vi "恢复参数.vi"(8 "仪器公式":T2(array[cluster]), 9 "量程参数":T3(array[cluster]), 10 "试剂容量参数":T4, 11 "外设参数":cluster{"仪器版本":T1, "error out":errorcluster}) -> (3 "恢复结果":string)   [LabVIEW 2022 SP3, in "斯坦道总氮.lvlib"]
uses:
  <vilib>/NI/Progress Bar/Progress Bar.lvlib
  <vilib>/Utility/config.llb/NI_LVConfig.lvlib
  <userlib>/_OpenG.lib/variantconfig/variantconfig.llb/openg_variant_configuration_file.lvlib
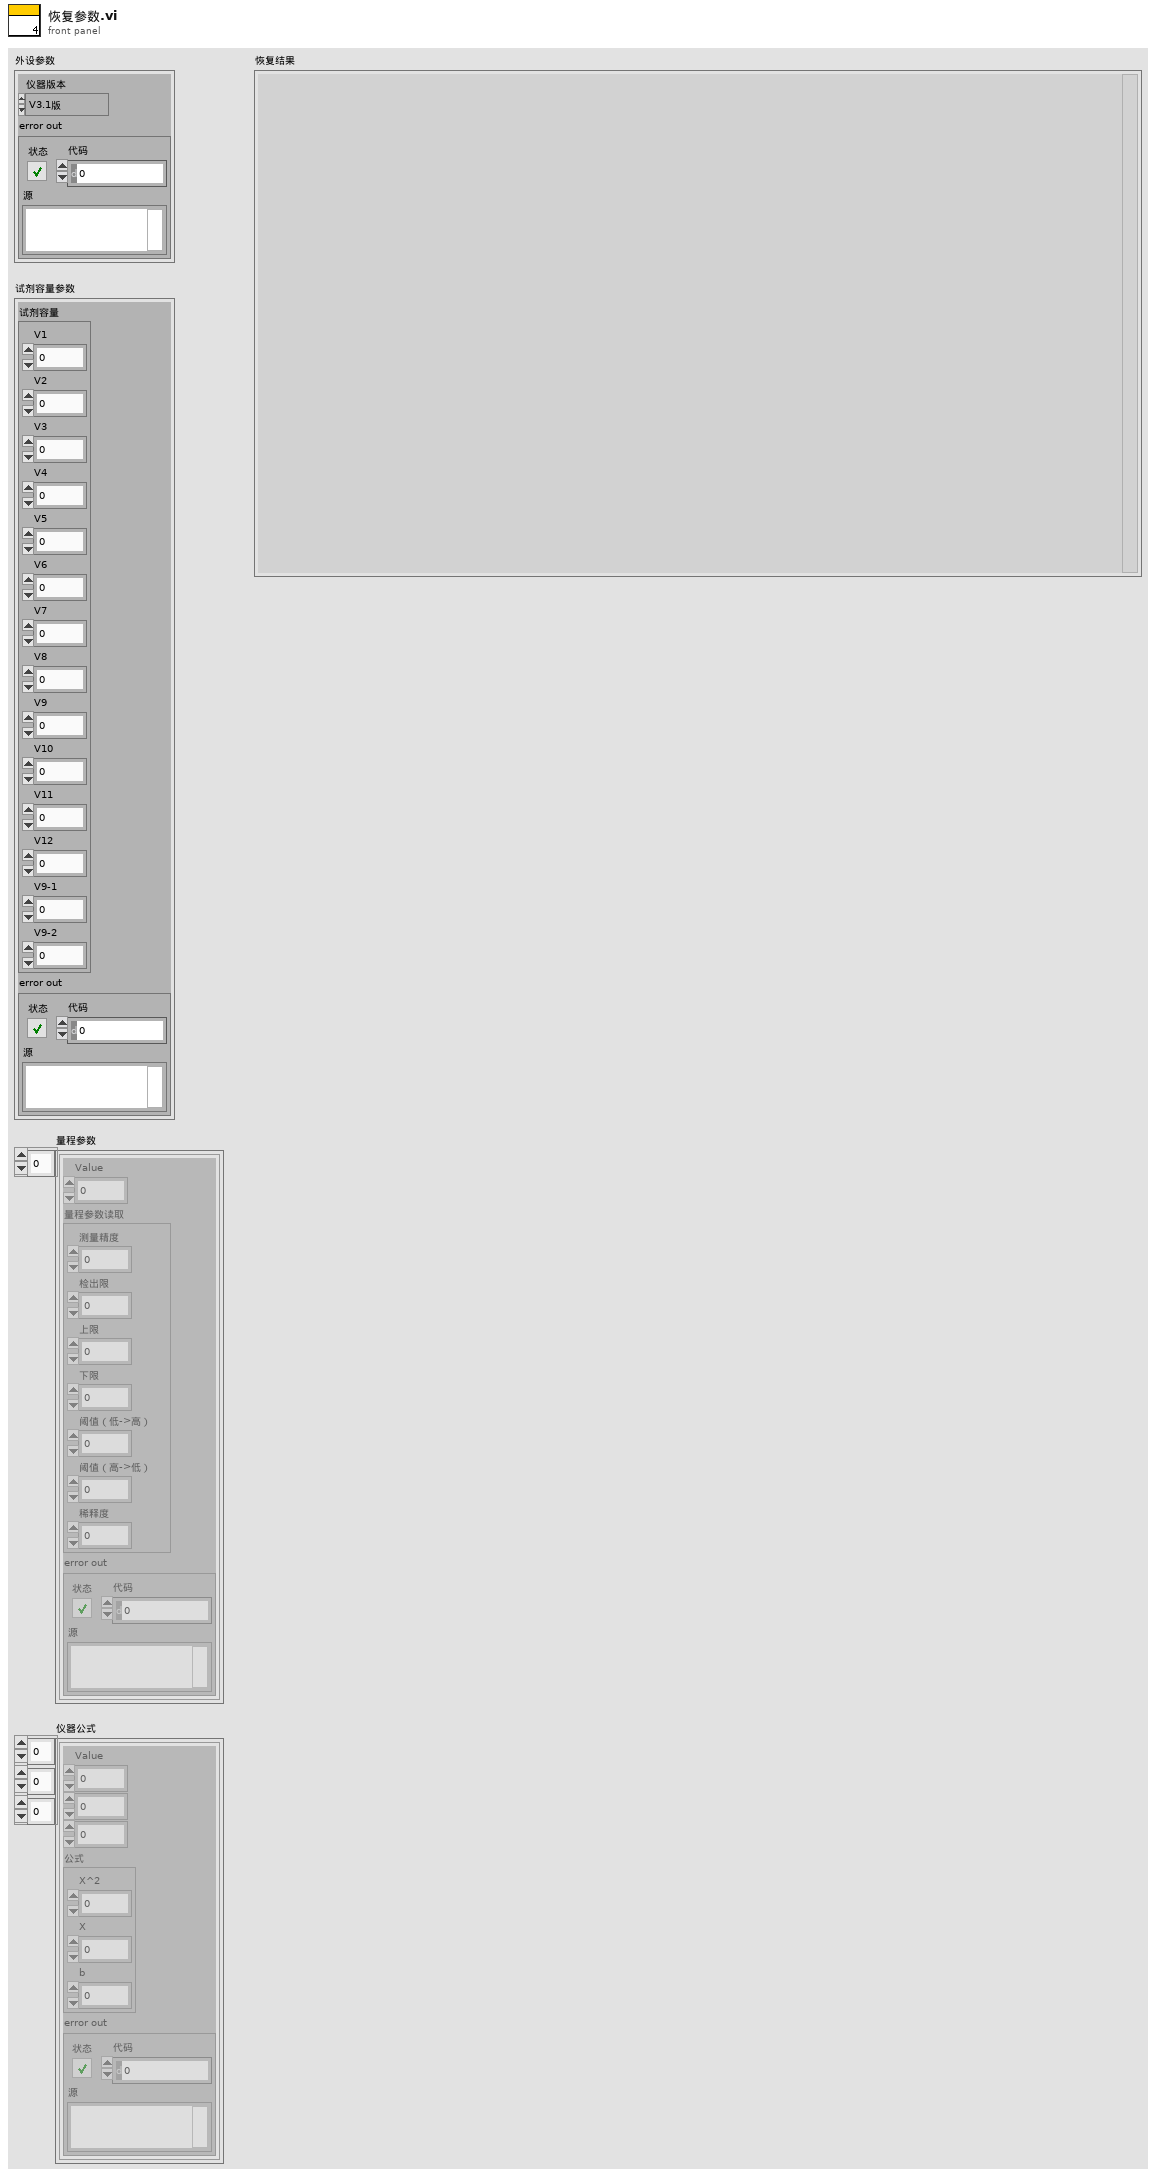
[diagram p1: front panel]
types:
  T1 = typedef "SingleStepTestV3.lvlib/SingleStepTestV3.lvclass/仪器版本.ctl" = enum16{"V3.1版", "V4版", "V3版", "V4.2版"}
  T2 = cluster{"Value":u16, i32, i32, "公式":cluster{"X^2":dbl, "X":dbl, "b":dbl}, "error out":errorcluster}[][][]
  T3 = cluster{"Value":u16, "量程参数读取":cluster{"测量精度":u16, "检出限":dbl, "上限":dbl, "下限":dbl, "阈值（低->高）":dbl, "阈值（高->低）":dbl, "稀释度":dbl}, "error out":errorcluster}[]
  T4 = cluster{"试剂容量":cluster{"V1":sgl, "V2":sgl, "V3":sgl, "V4":sgl, "V5":sgl, "V6":sgl, "V7":sgl, "V8":sgl, "V9":sgl, "V10":sgl, "V11":sgl, "V12":sgl, "V9-1":sgl, "V9-2":sgl}, "error out":errorcluster}
  T5 = enum16{"恢复外设参数", "恢复试剂容量参数", "恢复量程参数", "恢复仪器公式", "结束"}
  T6 = typedef "NI_LVConfig.lvlib/Config Data RefNum.ctl" = refnum<k1>
  T7 = typedef "斯坦道总氮.lvlib/V3.1版外设参数.ctl" = cluster{"泵类型":u8, "进样速度":u32, "出样速度":u32, "泵阀量":u8, "阀方向":u8, "光谱仪类型":u8, "光谱采样次数":u8, "氙灯次数":u8, "B":u16, "C":u16, "D":u16, "E":u16, "B_COD":u16, "C_COD":u16, "D_COD":u16, "E_COD":u16, "G":u16, "M":u16, "N":u16, "氨氮注射泵控温下限":sgl, "氨氮注射泵控温上限":sgl, "总氮注射泵控温下限":sgl, "总氮注射泵控温上限":sgl, "消解温度下限":sgl, "消解温度上限":sgl, "加热10s限值":sgl, "KP":sgl, "KI":sgl, "KD":sgl, "高温高压阀开阀温度":sgl, "总氮x公式0":u8, "总氮x公式1":sgl, "总氮x公式2":sgl, "总磷浊度稀释系数":sgl, "总磷浊度补偿权重1":sgl, "总磷浊度补偿权重2":sgl, "盐度系数":sgl, "氨氮补偿系数1":sgl, "氨氮补偿系数2":sgl}
  T8 = typedef "斯坦道总氮.lvlib/V4版外设参数.ctl" = cluster{"泵类型":u8, "注射泵正常速度":u32, "注射泵慢速":u32, "阀型号":u8, "res":u8, "光谱仪类型":u8, "光谱采样次数":u8, "氙灯次数":u8, "B":u16, "C":u16, "D":u16, "E":u16, "B_COD":u16, "C_COD":u16, "D_COD":u16, "E_COD":u16, "G":u16, "M":u16, "N":u16, "降温下限":sgl, "降温上限":sgl, "恒温温度下限":sgl, "恒温温度上限":sgl, "消解温度下限":sgl, "消解温度上限":sgl, "加热10s限值":sgl, "KP":sgl, "KI":sgl, "KD":sgl, "高温高压阀开阀温度":sgl, "总氮x公式0":u8, "总氮x公式1":sgl, "总氮x公式2":sgl, "总磷浊度稀释系数":sgl, "总磷浊度补偿权重1":sgl, "总磷浊度补偿权重2":sgl, "盐度系数":sgl, "氨氮补偿系数1":sgl, "氨氮补偿系数2":sgl, "缺试剂传感器阈值":u16}
  T9 = typedef "斯坦道总氮.lvlib/V3版外设参数.ctl" = cluster{"泵类型":u8, "进样速度":u32, "出样速度":u32, "泵阀量":u8, "光谱仪类型":u8, "光谱采样次数":u8, "氙灯次数":u8, "B":u16, "C":u16, "D":u16, "E":u16, "B_COD":u16, "C_COD":u16, "D_COD":u16, "E_COD":u16, "G":u16, "M":u16, "N":u16, "氨氮注射泵控温下限":sgl, "氨氮注射泵控温上限":sgl, "总氮注射泵控温下限":sgl, "总氮注射泵控温上限":sgl, "消解温度下限":sgl, "消解温度上限":sgl, "加热10s限值":sgl, "高温高压阀开阀温度":sgl, "总氮x公式0":u8, "总氮x公式1":sgl, "总氮x公式2":sgl, "总磷浊度稀释系数":sgl, "总磷浊度补偿权重1":sgl, "总磷浊度补偿权重2":sgl, "盐度系数":sgl, "氨氮补偿系数1":sgl, "氨氮补偿系数2":sgl}
  T10 = typedef "斯坦道总氮.lvlib/V4.2版外设参数.ctl" = cluster{"工作模式":u16, "泵类型":u16, "阀型号":u16, "注射泵进样速度":u16, "注射泵出样速度":u16, "注射泵滴定速度":u16, "res":u16, "注射泵慢速":u16, "光谱仪类型":u16, "光谱采样次数":u16, "氙灯次数":u16, "B":u16, "C":u16, "D":u16, "E":u16, "B_COD":u16, "C_COD":u16, "D_COD":u16, "E_COD":u16, "G":u16, "M":u16, "N":u16, "温度校准参数":sgl, "降温温度":sgl, "恒温温度":sgl, "消解温度":sgl, "高温高压阀开阀温度":sgl, "加热超时时间":sgl, "KP":sgl, "KI":sgl, "KD":sgl, "消解PID积分上限":sgl, "恒温PID积分上限":sgl, "PID积分下限":sgl, "缺试剂传感器阈值":u16, "滴定延时":u16, "滴定斜率阈值":sgl, "总氮x公式0":u16, "总氮x公式1":sgl, "总氮x公式2":sgl, "总磷浊度稀释系数":sgl, "总磷浊度补偿权重1":sgl, "总磷浊度补偿权重2":sgl, "盐度系数":sgl, "氨氮补偿系数1":sgl, "氨氮补偿系数2":sgl}
  T11 = cluster{"V1":sgl, "V2":sgl, "V3":sgl, "V4":sgl, "V5":sgl, "V6":sgl, "V7":sgl, "V8":sgl, "V9":sgl, "V10":sgl, "V11":sgl, "V12":sgl, "V9-1":sgl, "V9-2":sgl}
  T12 = cluster{"测量精度":u16, "检出限":dbl, "上限":dbl, "下限":dbl, "阈值（低->高）":dbl, "阈值（高->低）":dbl, "稀释度":dbl}
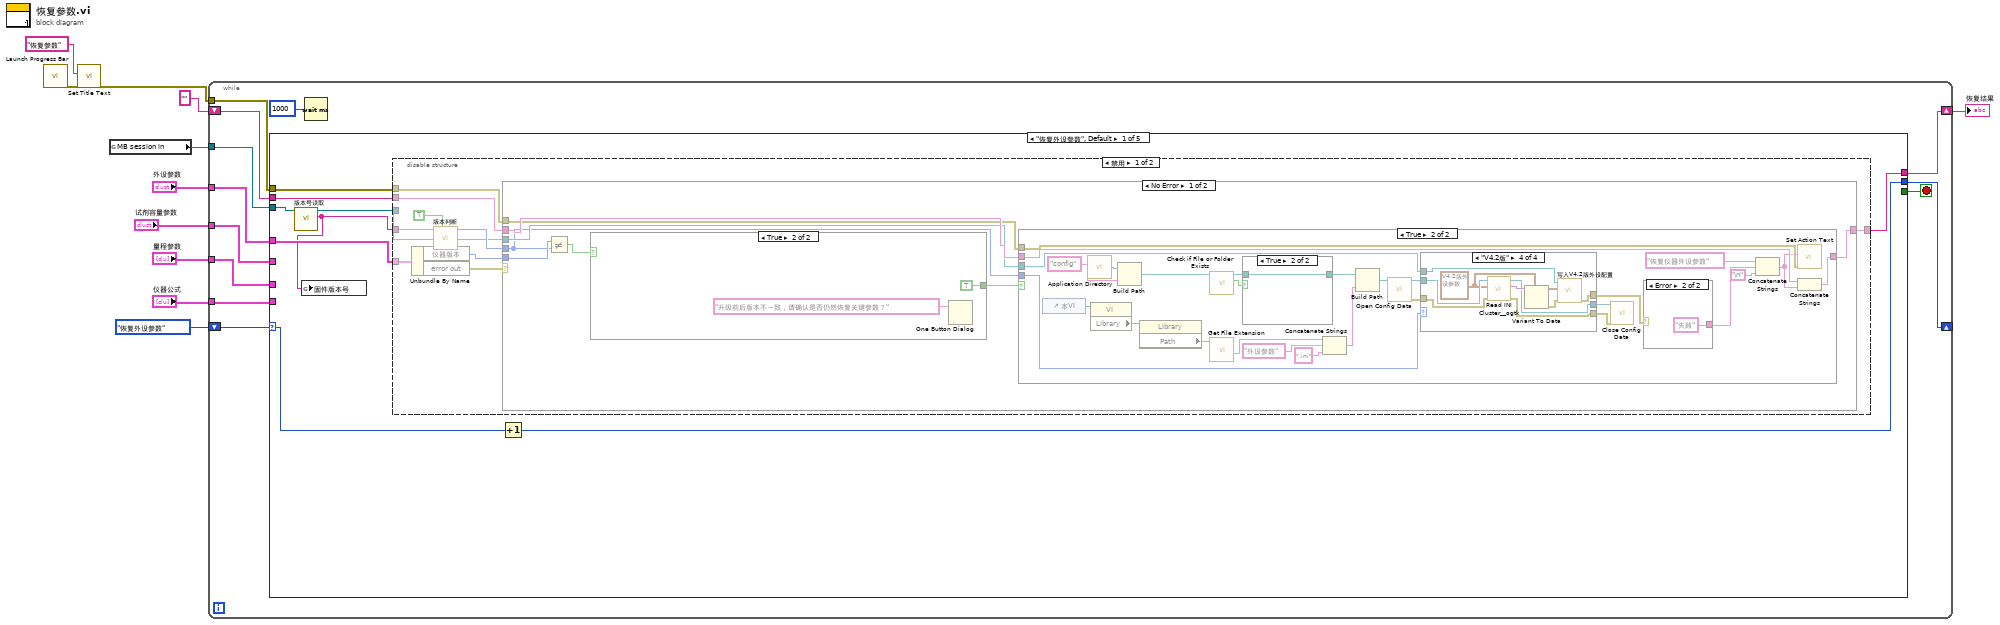
[diagram p0: block diagram]
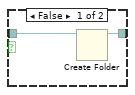
[diagram p3: hidden frame]
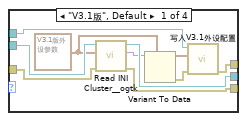
[diagram p4: hidden frame]
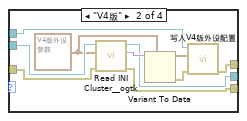
[diagram p5: hidden frame]
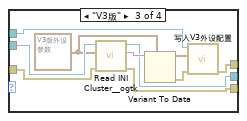
[diagram p6: hidden frame]
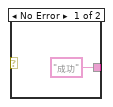
[diagram p7: hidden frame]
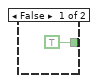
[diagram p8: hidden frame]
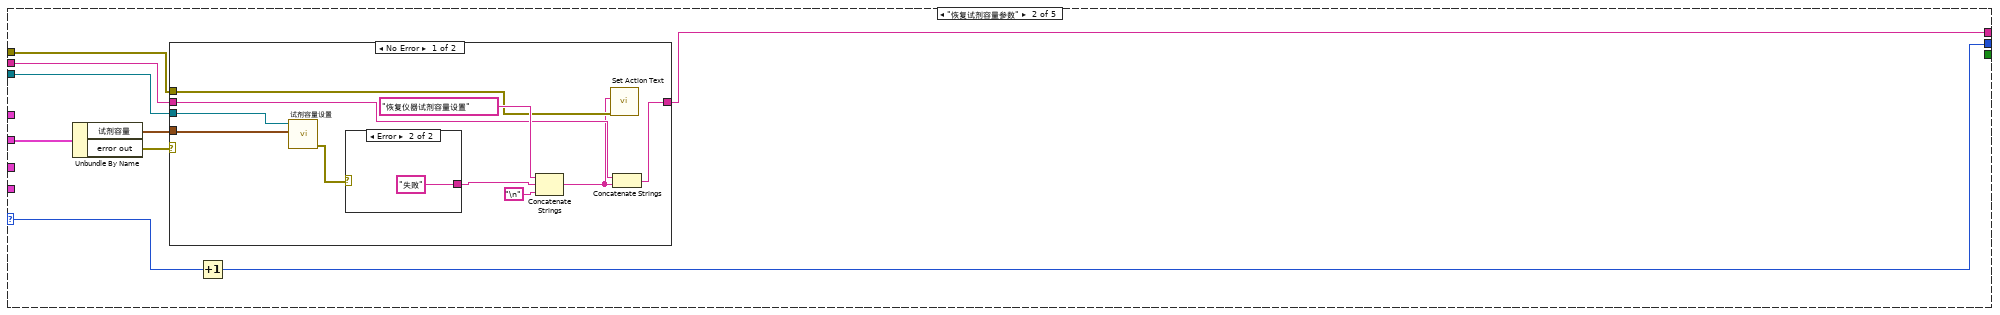
[diagram p11: hidden frame]
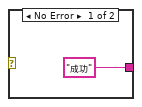
[diagram p12: hidden frame]
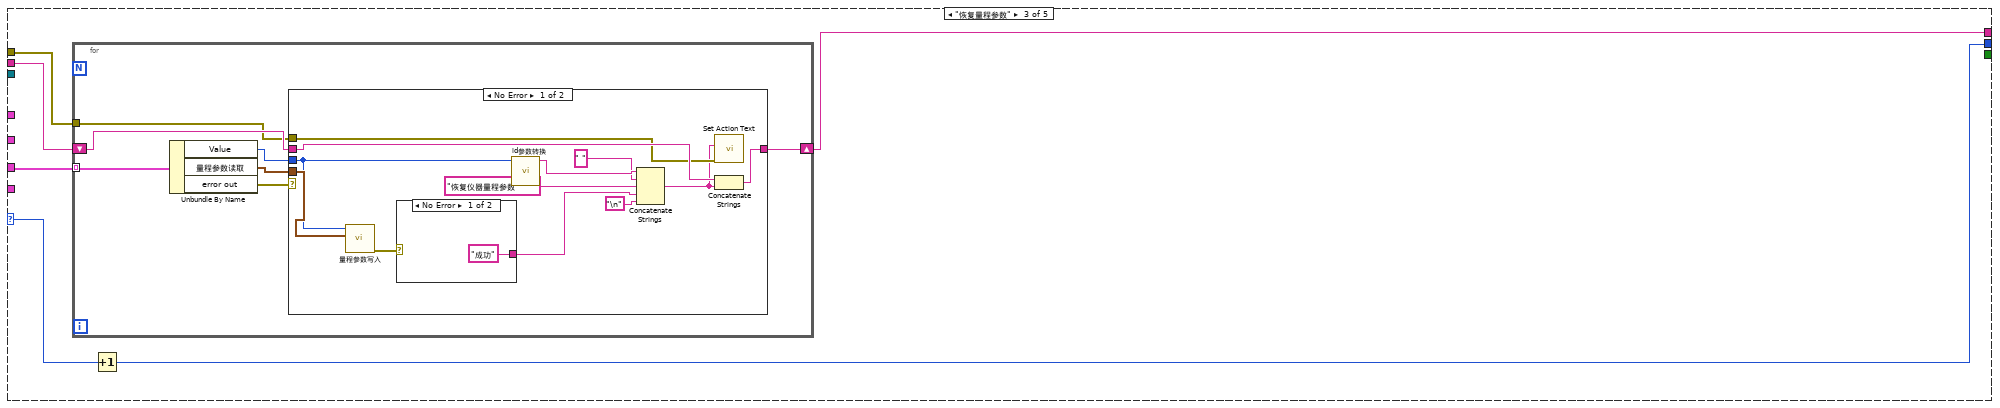
[diagram p14: hidden frame]
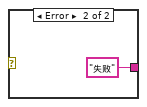
[diagram p15: hidden frame]
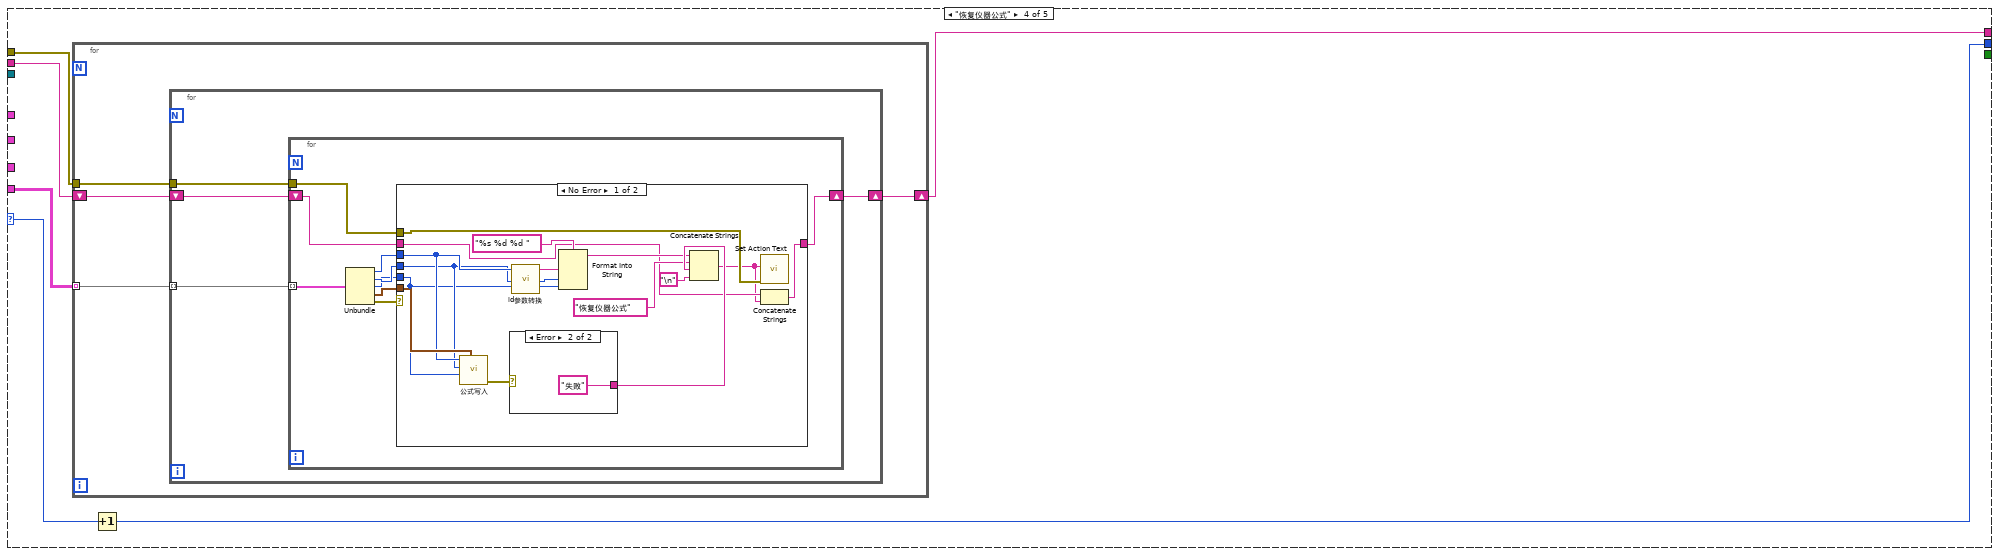
[diagram p17: hidden frame]
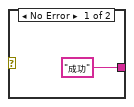
[diagram p18: hidden frame]
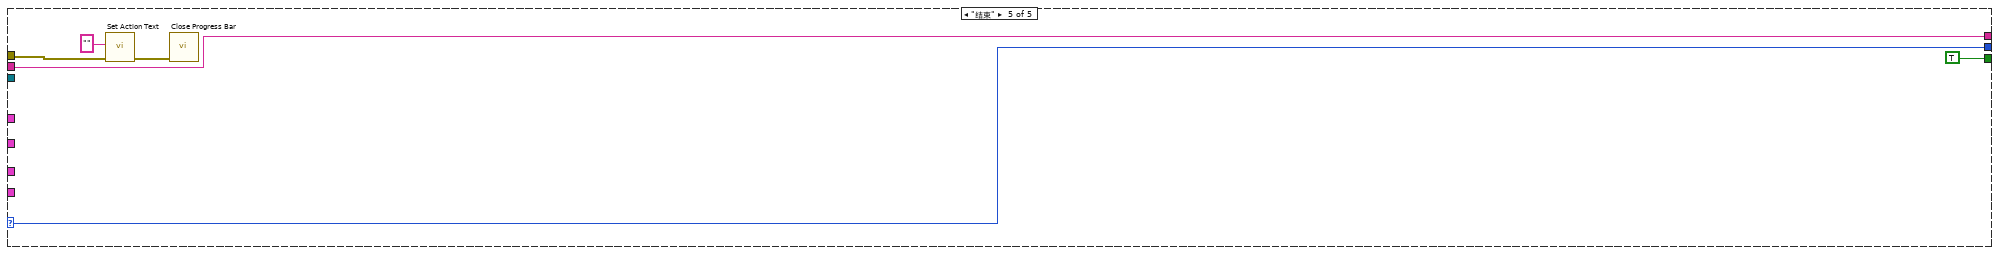
[diagram p20: hidden frame]
diagram:
  n1 = call <vilib>:"Launch Progress Bar.vi"() -> ("error out"=w4:errorcluster)  [unwired: 10 in, 1 out]
  n2 = call <vilib>:"Set Title Text.vi"("error in (no error)"=w4, "Installer Title"="恢复参数") -> ("error out"=w3:errorcluster)  [unwired: 9 in]
  n3 = global read "VAR总磷总氮全局变量.vi" "MB session in"() -> (w9:refnum<class "MB_Master.lvclass">)
  n4 = while {
    shift-right: [w22] -> _
    shift-left: T5."恢复外设参数" ("枚举") -> [w23]
    tunnel: "外设参数" -> [w21]
    shift-right: [w15] -> w5
    shift-left: "" -> [w20]
    tunnel: w9 -> [w19]
    tunnel: "试剂容量参数" -> [w18]
    tunnel: "量程参数" -> [w17]
    tunnel: "仪器公式" -> [w16]
    tunnel: w3 -> [w13]
    stop <- w14 stop-if-true
    n5 = case shown="\"恢复外设参数\", Default" w23 {
      selector: w23 -> [w32 w137 w156 w184 w225]
      tunnel: [w31 w136 w155 w183 w225] -> w22
      tunnel: w21 -> [w27 _ _ _ _]
      tunnel: w20 -> [w30 w131 w153 w181 w224]
      tunnel: w19 -> [w26 w133 _ _ _]
      tunnel: w18 -> [_ w135 _ _ _]
      tunnel: w17 -> [_ _ w154 _ _]
      tunnel: w16 -> [_ _ _ w182 _]
      tunnel: [w29 w130 w152 w180 w224] -> w15
      tunnel: [_ _ _ _ TRUE] -> w14
      tunnel: w13 -> [w28 w129 w151 w179 w222]
      frame "恢复外设参数", Default {
        n6 = call "版本号读取.vi"("MB session in"=w26) -> ("固件版本号"=w24:string, "MB session out"=w25:refnum<class "MB_Master.lvclass">)  [unwired: 8 in, 1 out]
        n7 = global write "VAR总磷总氮全局变量.vi" "固件版本号"(w24) -> ()
        n8 = disable-structure shown="禁用" {
          disable-tunnel: w30 -> [w42 _]
          disable-tunnel: [w41 _] -> w29
          disable-tunnel: w28 -> [w40 _]
          disable-tunnel: w27 -> [w39 _]
          disable-tunnel: w25 -> [w36 _]
          disable-tunnel: w24 -> [w33 _]
          frame Disabled {
            n9 = Unbundle By Name(w39) -> ("仪器版本"=w34:T1, "error out"=w38:errorcluster)
            n10 = call "版本判断.vi"("Extern"=TRUE, "固件版本号"=w33) -> ("仪器版本"=w37:T1)  [unwired: 9 in]
            n11 = case shown="No Error" w38 {
              tunnel: w36 -> [w47 _]
              tunnel: w37 -> [w45 _]
              tunnel: [w49 w128] -> w41
              tunnel: w42 -> [w50 w128]
              tunnel: w40 -> [w48 _]
              tunnel: w34 -> [w46 _]
              frame No Error {
                n12 = Not Equal?(x=w46, y=w45) -> (x != y?=w44:bool)
                n13 = case shown="True" w44 {
                  tunnel: [TRUE ("T button?") TRUE ("T button?")] -> w43
                  frame False {
                  }
                  frame True {
                    n14 = One Button Dialog(message="升级前后版本不一致，请确认是否仍然恢复关键参数？" ("消息")) -> ()  [unwired: 1 in, 1 out]
                  }
                }
                n15 = case shown="True" w43 {
                  tunnel: w50 -> [w51 w76]
                  tunnel: [w51 w75] -> w49
                  tunnel: w48 -> [_ w74]
                  tunnel: w47 -> [_ w71]
                  tunnel: w45 -> [_ w57]
                  frame False {
                  }
                  frame True {
                    n16 = control-ref of="本VI"() -> (w70:refnum<vi>)
                    n17 = call <vilib>:"Application Directory.vi"() -> ("Application Directory"=w60:path)
                    n18 = property class="VI"(reference=w70) -> ("Library"=w58:refnum<vi>)  [unwired: 1 in, 2 out]
                    n19 = Build Path(base path=w60, name or relative path="config" ("名称或相对路径")) -> (appended path=w62:path)
                    n20 = property class="Library"(reference=w58) -> ("Path"=w59:path)  [unwired: 1 in, 2 out]
                    n21 = call <vilib>:"Check if File or Folder Exists.vi"("path"=w62) -> ("file or folder exists?"=w65:bool, "dup path"=w66:path)  [unwired: 8 in, 1 out]
                    n22 = call <vilib>:"Get File Extension.vi"("file"=w59) -> ("filename without extension"=w68:string)  [unwired: 6 in, 4 out]
                    n23 = case shown="True" w65 {
                      tunnel: w66 -> [w81 w82]
                      tunnel: [w80 w82] -> w67
                      frame False {
                        n24 = Create Folder(path (use dialog)=w81) -> (created path=w80:path)  [unwired: 2 in, 2 out]
                      }
                      frame True {
                      }
                    }
                    n25 = Concatenate Strings(w68, "外设参数" ("字符串"), ".ini" ("字符串")) -> (w64:string)
                    n26 = Build Path(base path=w67, name or relative path=w64) -> (appended path=w56:path)
                    n27 = call <vilib>:"Open Config Data.vi"("configuration file path"=w56) -> ("error out"=w54:errorcluster, "refnum"=w55:T6)  [unwired: 8 in, 1 out]
                    n28 = case shown="\"V4.2版\"" w57 {
                      tunnel: [w92 w101 w111 w121] -> w72
                      tunnel: w71 -> [w91 w102 w112 w122]
                      tunnel: w55 -> [w90 w99 w109 w119]
                      tunnel: w54 -> [w89 w98 w108 w118]
                      tunnel: [w88 w96 w106 w116] -> w53
                      tunnel: [w87 w97 w107 w117] -> w52
                      frame "V3.1版", Default {
                        w83 = T7 {"泵类型"=0, "进样速度"=0, "出样速度"=0, "泵阀量"=0, "阀方向"=0, "光谱仪类型"=0, "光谱采样次数"=0, "氙灯次数"=0, "B"=0, "C"=0, "D"=0, "E"=0, "B_COD"=0, "C_COD"=0, "D_COD"=0, "E_COD"=0, "G"=0, "M"=0, "N"=0, "氨氮注射泵控温下限"=0.0, "氨氮注射泵控温上限"=0.0, "总氮注射泵控温下限"=0.0, "总氮注射泵控温上限"=0.0, "消解温度下限"=0.0, "消解温度上限"=0.0, "加热10s限值"=0.0, "KP"=52.0, "KI"=1.156, "KD"=800.0, "高温高压阀开阀温度"=0.0, "总氮x公式0"=0, "总氮x公式1"=0.0, "总氮x公式2"=0.0, "总磷浊度稀释系数"=0.0, "总磷浊度补偿权重1"=0.0, "总磷浊度补偿权重2"=0.0, "盐度系数"=0.0, "氨氮补偿系数1"=0.0, "氨氮补偿系数2"=0.0} ("外设配置")
                        n29 = call <userlib>:"Read INI Cluster__ogtk.vi"("error in (no error)"=w89, "INI Fomatted Cluster Type"=w83, "refnum"=w90) -> ("error out"=w88:errorcluster, "INI Fomatted Cluster"=w86:variant, "dup refnum"=w87:T6)  [unwired: 4 in, 2 out]
                        n30 = Variant To Data(type=w83, Variant=w86) -> (data=w85:T7, error out=w84:errorcluster)  [unwired: 1 in]
                        n31 = call "写入V3.1外设配置.vi"("error in (no error)"=w84, "外设配置"=w85, "MB session in"=w91) -> ("error out"=w92:errorcluster)  [unwired: 7 in, 1 out]
                      }
                      frame "V4版" {
                        w93 = T8 {"泵类型"=0, "注射泵正常速度"=0, "注射泵慢速"=0, "阀型号"=0, "res"=0, "光谱仪类型"=0, "光谱采样次数"=0, "氙灯次数"=0, "B"=0, "C"=0, "D"=0, "E"=0, "B_COD"=0, "C_COD"=0, "D_COD"=0, "E_COD"=0, "G"=0, "M"=0, "N"=0, "降温下限"=0.0, "降温上限"=0.0, "恒温温度下限"=0.0, "恒温温度上限"=0.0, "消解温度下限"=0.0, "消解温度上限"=0.0, "加热10s限值"=0.0, "KP"=0.0, "KI"=0.0, "KD"=0.0, "高温高压阀开阀温度"=0.0, "总氮x公式0"=0, "总氮x公式1"=0.0, "总氮x公式2"=0.0, "总磷浊度稀释系数"=0.0, "总磷浊度补偿权重1"=0.0, "总磷浊度补偿权重2"=0.0, "盐度系数"=0.0, "氨氮补偿系数1"=0.0, "氨氮补偿系数2"=0.0, "缺试剂传感器阈值"=0} ("外设配置")
                        n32 = call <userlib>:"Read INI Cluster__ogtk.vi"("error in (no error)"=w98, "INI Fomatted Cluster Type"=w93, "refnum"=w99) -> ("error out"=w96:errorcluster, "INI Fomatted Cluster"=w100:variant, "dup refnum"=w97:T6)  [unwired: 4 in, 2 out]
                        n33 = Variant To Data(type=w93, Variant=w100) -> (data=w95:T8, error out=w94:errorcluster)  [unwired: 1 in]
                        n34 = call "写入V4版外设配置.vi"("error in (no error)"=w94, "外设配置"=w95, "MB session in"=w102) -> ("error out"=w101:errorcluster)  [unwired: 7 in, 1 out]
                      }
                      frame "V3版" {
                        w103 = T9 {"泵类型"=0, "进样速度"=0, "出样速度"=0, "泵阀量"=0, "光谱仪类型"=0, "光谱采样次数"=0, "氙灯次数"=0, "B"=0, "C"=0, "D"=0, "E"=0, "B_COD"=0, "C_COD"=0, "D_COD"=0, "E_COD"=0, "G"=0, "M"=0, "N"=0, "氨氮注射泵控温下限"=0.0, "氨氮注射泵控温上限"=0.0, "总氮注射泵控温下限"=0.0, "总氮注射泵控温上限"=0.0, "消解温度下限"=0.0, "消解温度上限"=0.0, "加热10s限值"=0.0, "高温高压阀开阀温度"=0.0, "总氮x公式0"=0, "总氮x公式1"=0.0, "总氮x公式2"=0.0, "总磷浊度稀释系数"=0.0, "总磷浊度补偿权重1"=0.0, "总磷浊度补偿权重2"=0.0, "盐度系数"=0.0, "氨氮补偿系数1"=0.0, "氨氮补偿系数2"=0.0} ("外设配置")
                        n35 = call <userlib>:"Read INI Cluster__ogtk.vi"("error in (no error)"=w108, "INI Fomatted Cluster Type"=w103, "refnum"=w109) -> ("error out"=w106:errorcluster, "INI Fomatted Cluster"=w110:variant, "dup refnum"=w107:T6)  [unwired: 4 in, 2 out]
                        n36 = Variant To Data(type=w103, Variant=w110) -> (data=w105:T9, error out=w104:errorcluster)  [unwired: 1 in]
                        n37 = call "写入V3外设配置.vi"("error in (no error)"=w104, "外设配置"=w105, "MB session in"=w112) -> ("error out"=w111:errorcluster)  [unwired: 7 in, 1 out]
                      }
                      frame "V4.2版" {
                        w113 = T10 {"工作模式"=0, "泵类型"=0, "阀型号"=0, "注射泵进样速度"=0, "注射泵出样速度"=0, "注射泵滴定速度"=0, "res"=0, "注射泵慢速"=0, "光谱仪类型"=0, "光谱采样次数"=0, "氙灯次数"=0, "B"=0, "C"=0, "D"=0, "E"=0, "B_COD"=0, "C_COD"=0, "D_COD"=0, "E_COD"=0, "G"=0, "M"=0, "N"=0, "温度校准参数"=0.0, "降温温度"=0.0, "恒温温度"=0.0, "消解温度"=0.0, "高温高压阀开阀温度"=0.0, "加热超时时间"=0.0, "KP"=0.0, "KI"=0.0, "KD"=0.0, "消解PID积分上限"=0.0, "恒温PID积分上限"=0.0, "PID积分下限"=0.0, "缺试剂传感器阈值"=0, "滴定延时"=0, "滴定斜率阈值"=0.0, "总氮x公式0"=0, "总氮x公式1"=0.0, "总氮x公式2"=0.0, "总磷浊度稀释系数"=0.0, "总磷浊度补偿权重1"=0.0, "总磷浊度补偿权重2"=0.0, "盐度系数"=0.0, "氨氮补偿系数1"=0.0, "氨氮补偿系数2"=0.0} ("外设配置")
                        n38 = call <userlib>:"Read INI Cluster__ogtk.vi"("error in (no error)"=w118, "INI Fomatted Cluster Type"=w113, "refnum"=w119) -> ("error out"=w116:errorcluster, "INI Fomatted Cluster"=w120:variant, "dup refnum"=w117:T6)  [unwired: 4 in, 2 out]
                        n39 = Variant To Data(type=w113, Variant=w120) -> (data=w115:T10, error out=w114:errorcluster)  [unwired: 1 in]
                        n40 = call "写入V4.2版外设配置.vi"("error in (no error)"=w114, "外设配置"=w115, "MB session in"=w122) -> ("error out"=w121:errorcluster)  [unwired: 7 in, 1 out]
                      }
                    }
                    n41 = call <vilib>:"Close Config Data.vi"("error in (no error)"=w53, "refnum"=w52) -> ()  [unwired: 8 in, 2 out]
                    n42 = case shown="Error" w72 {
                      tunnel: ["成功" "失败"] -> w78
                      frame No Error {
                      }
                      frame Error {
                      }
                    }
                    n43 = Concatenate Strings("恢复仪器外设参数" ("字符串"), w78, "\n") -> (w73:string)
                    n44 = call <vilib>:"Set Action Text.vi"("error in (no error)"=w74, "Action Text"=w73) -> ()  [unwired: 9 in, 1 out]
                    n45 = Concatenate Strings(w76, w73) -> (w75:string)
                  }
                }
              }
              frame Error {
              }
            }
          }
          frame Enabled {
          }
        }
        n46 = Increment(x=w32) -> (x+1=w31:T5)
      }
      frame "恢复试剂容量参数" {
        n47 = Unbundle By Name(w135) -> ("试剂容量"=w134:T11, "error out"=w132:errorcluster)
        n48 = case shown="No Error" w132 {
          tunnel: w134 -> [w147 _]
          tunnel: w133 -> [w146 _]
          tunnel: w131 -> [w141 w150]
          tunnel: [w140 w150] -> w130
          tunnel: w129 -> [w139 _]
          frame No Error {
            n49 = call "试剂容量设置.vi"("试剂容量"=w147, "MB session in"=w146) -> ("error out"=w143:errorcluster)  [unwired: 8 in, 1 out]
            n50 = case shown="Error" w143 {
              tunnel: ["成功" "失败"] -> w144
              frame No Error {
              }
              frame Error {
              }
            }
            n51 = Concatenate Strings("恢复仪器试剂容量设置" ("字符串"), w144, "\n") -> (w138:string)
            n52 = call <vilib>:"Set Action Text.vi"("error in (no error)"=w139, "Action Text"=w138) -> ()  [unwired: 9 in, 1 out]
            n53 = Concatenate Strings(w141, w138) -> (w140:string)
          }
          frame Error {
          }
        }
        n54 = Increment(x=w137) -> (x+1=w136:T5)
      }
      frame "恢复量程参数" {
        n55 = for {
          tunnel: w154 -> [w163] mode=indexing
          shift-right: [w158] -> w152
          shift-left: w153 -> [w159]
          tunnel: w151 -> [w157]
          n56 = Unbundle By Name(w163) -> ("Value"=w161:u16, "量程参数读取"=w162:T12, "error out"=w160:errorcluster)
          n57 = case shown="No Error" w160 {
            tunnel: w162 -> [w175 _]
            tunnel: w161 -> [w171 _]
            tunnel: w159 -> [w167 w178]
            tunnel: [w166 w178] -> w158
            tunnel: w157 -> [w165 _]
            frame No Error {
              n58 = call "量程参数写入.vi"("量程参数写入"=w175, "测量参数"=w171) -> ("error out"=w172:errorcluster)  [unwired: 8 in]
              n59 = case shown="No Error" w172 {
                tunnel: ["成功" "失败"] -> w173
                frame No Error {
                }
                frame Error {
                }
              }
              n60 = call "id参数转换.vi"("id"=w171) -> ("table输出"=w170:string)  [unwired: 9 in, 1 out]
              n61 = Concatenate Strings(w170, " " ("字符串"), "恢复仪器量程参数" ("字符串"), w173, "\n") -> (w164:string)
              n62 = call <vilib>:"Set Action Text.vi"("error in (no error)"=w165, "Action Text"=w164) -> ()  [unwired: 9 in, 1 out]
              n63 = Concatenate Strings(w167, w164) -> (w166:string)
            }
            frame Error {
            }
          }
        }
        n64 = Increment(x=w156) -> (x+1=w155:T5)
      }
      frame "恢复仪器公式" {
        n65 = for {
          tunnel: w182 -> [w188] mode=indexing
          shift-right: [w186] -> w180
          shift-left: w181 -> [w187]
          tunnel: w179 -> [w185]
          n66 = for {
            tunnel: w188 -> [w192] mode=indexing
            shift-right: [w190] -> w186
            shift-left: w187 -> [w191]
            tunnel: w185 -> [w189]
            n67 = for {
              tunnel: w192 -> [w201] mode=indexing
              shift-right: [w194] -> w190
              shift-left: w191 -> [w195]
              tunnel: w189 -> [w193]
              n68 = Unbundle(w201) -> ("Value"=w199:u16, w198:i32, w197:i32, "公式"=w196:cluster{"X^2":dbl, "X":dbl, "b":dbl}, "error out"=w200:errorcluster)
              n69 = case shown="No Error" w200 {
                tunnel: w199 -> [w209 _]
                tunnel: w198 -> [w208 _]
                tunnel: w197 -> [w207 _]
                tunnel: w196 -> [w216 _]
                tunnel: w195 -> [w205 w219]
                tunnel: [w204 w219] -> w194
                tunnel: w193 -> [w203 _]
                frame No Error {
                  n70 = call "公式写入.vi"("公式"=w216, "量程"=w207, "测量模式"=w208, "测量参数"=w209) -> ("error out"=w210:errorcluster)  [unwired: 7 in]
                  n71 = case shown="Error" w210 {
                    tunnel: ["成功" "失败"] -> w215
                    frame No Error {
                    }
                    frame Error {
                    }
                  }
                  n72 = call "id参数转换.vi"("id"=w209) -> ("table输出"=w212:string)  [unwired: 9 in, 1 out]
                  n73 = Format Into String(format string="%s %d %d " ("格式字符串"), w212, w208, w207) -> (resulting string=w211:string)  [unwired: 2 in, 1 out]
                  n74 = Concatenate Strings(w211, "恢复仪器公式" ("字符串"), w215, "\n") -> (w202:string)
                  n75 = call <vilib>:"Set Action Text.vi"("error in (no error)"=w203, "Action Text"=w202) -> ()  [unwired: 9 in, 1 out]
                  n76 = Concatenate Strings(w205, w202) -> (w204:string)
                }
                frame Error {
                }
              }
            }
          }
        }
        n77 = Increment(x=w184) -> (x+1=w183:T5)
      }
      frame "结束" {
        n78 = call <vilib>:"Set Action Text.vi"("error in (no error)"=w222, "Action Text"="") -> ("error out"=w221:errorcluster)  [unwired: 9 in]
        n79 = call <vilib>:"Close Progress Bar.vi"("error in (no error)"=w221) -> ()  [unwired: 9 in, 2 out]
      }
    }
    n80 = Wait (ms)(milliseconds to wait=u32 1000 ("等待时间（毫秒）")) -> ()  [unwired: 1 out]
  }
  "恢复结果" <- w5
